vi "Auto settings.vi"(8 "error in (no error)":errorcluster, 10 "Assembly Tray Settings":T1, 11 "Assembly Tray in":refnum<class "Assembly Tray.lvclass">) -> (0 "error out":errorcluster, 3 "Assembly Tray out":refnum<class "Assembly Tray.lvclass">)   [LabVIEW 2021, in "Assembly Tray.lvclass"]
uses:
  Assembly Tray.lvclass
  C:/Users/HEP/Documents/GitHub/Gantry/UCSB-Gantry-HEP-main/Classes/Workspace/Fixture.lvclass
  Assembly Tray.lvclass/Assembly Tray.ctl
  Fixture.lvclass/Fixture.ctl
  Write Gantry Region.vi
  Write Position.vi
  Write Fixture ID.vi
  SubVIs/assembly_tray_region.vi
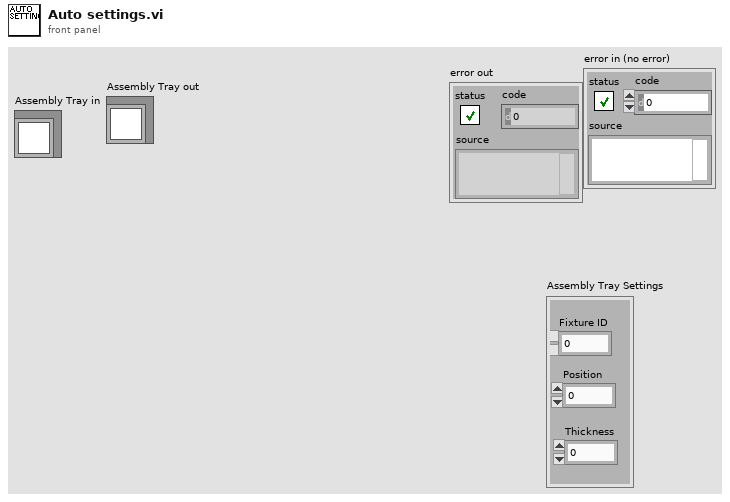
[diagram p1: front panel]
types:
  T1 = cluster{"Fixture ID":dbl, "Position":dbl, "Thickness":dbl}
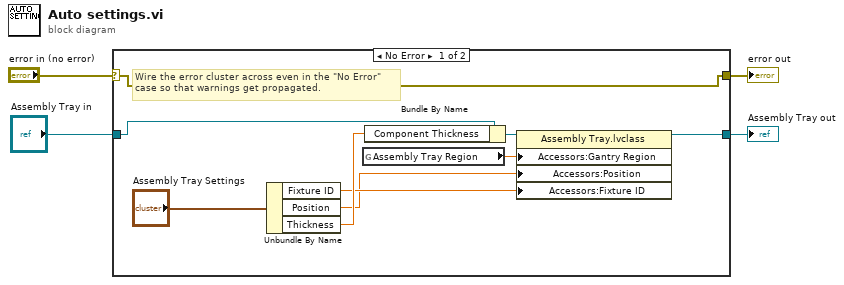
[diagram p0: block diagram]
diagram:
  n1 = case shown="No Error" "error in (no error)" {
    selector: "error in (no error)" -> [w13 w15]
    tunnel: [w13 w15] -> w3
    tunnel: [w12 w14] -> w1
    tunnel: "Assembly Tray in" -> [w11 w14]
    frame No Error {
      # "Wire the error cluster across even in the \"No Error\"\ncase so that warnings get propagated."
      n2 = Unbundle By Name("Assembly Tray Settings") -> ("Fixture ID"=w6:dbl, "Position"=w5:dbl, "Thickness"=w7:dbl)
      n3 = global read "assembly_tray_region.vi" "Assembly Tray Region"() -> (w9:dbl)
      n4 = Bundle By Name(cluster=w11, "Component Thickness"=w7) -> (w10:refnum<class "Assembly Tray.lvclass">)
      n5 = property class="Assembly Tray.lvclass"(reference=w10, "Accessors:Gantry Region"=w9, "Accessors:Position"=w5, "Accessors:Fixture ID"=w6) -> (reference out=w12:refnum<class "Assembly Tray.lvclass">)  [unwired: 1 in, 1 out]
    }
    frame Error {
    }
  }
  "error out" <- w3
  "Assembly Tray out" <- w1
